vi "Bundle Test Graph Data.vi"(6 "ia test data":T1, 7 "diam time array in":dbl[](array[numeric]), 8 "setpoint array in":dbl[](array[numeric]), 9 "force array in":dbl[](array[numeric]), 10 "force time array in":dbl[](array[numeric]), 11 "diam array in":dbl[](array[numeric])) -> (0 "setpoint array out":dbl[](array[numeric]), 1 "force array out":dbl[](array[numeric]), 2 "force time array out":dbl[](array[numeric]), 3 "diam array out":dbl[](array[numeric]), 5 "diam time array out":dbl[](array[numeric]))   [LabVIEW 2020]
uses:
  Inflation Test/Result Handling/Inflation Test Numeric Results.ctl
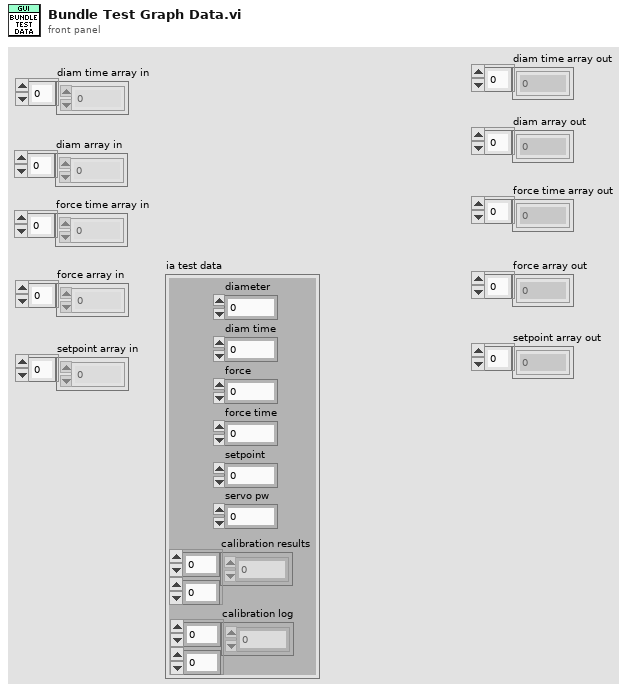
[diagram p1: front panel]
types:
  T1 = typedef "Inflation Test Numeric Results.ctl" = cluster{"diameter":dbl, "diam time":dbl, "force":dbl, "force time":dbl, "setpoint":dbl, "servo pw":dbl, "calibration log":dbl[][], "calibration results":dbl[][]}
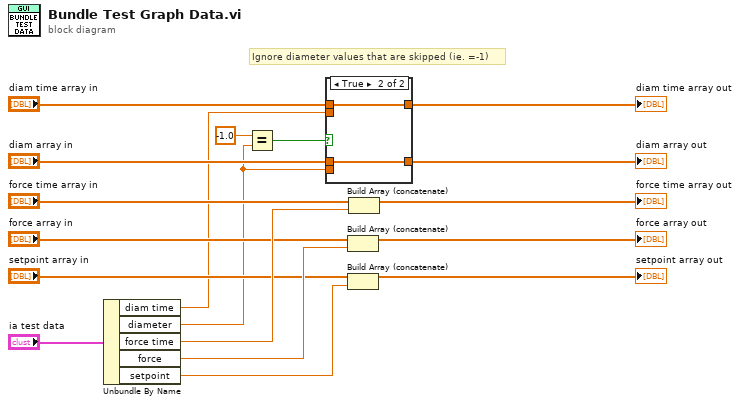
[diagram p0: block diagram]
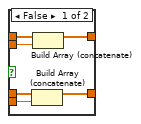
[diagram p2: hidden frame]
diagram:
  # "Ignore diameter values that are skipped (ie. =-1)"
  n1 = Unbundle By Name("ia test data") -> ("diam time"=w6:dbl, "diameter"=w3:dbl, "force time"=w11:dbl, "force"=w12:dbl, "setpoint"=w13:dbl)
  n2 = Equal?(x=-1.0, y=w3) -> (x = y?=w1:bool)
  n3 = case shown="True" w1 {
    tunnel: [w24 w25] -> w15
    tunnel: [w23 w26] -> w14
    tunnel: "diam array in" -> [w22 w25]
    tunnel: w6 -> [w21 _]
    tunnel: "diam time array in" -> [w20 w26]
    tunnel: w3 -> [w19 _]
    frame False {
      n4 = Build Array (concatenate)(w22, w19) -> (w24:dbl[])
      n5 = Build Array (concatenate)(w20, w21) -> (w23:dbl[])
    }
    frame True {
    }
  }
  "diam array out" <- w15
  "diam time array out" <- w14
  n6 = Build Array (concatenate)("force array in", w12) -> (→"force array out":dbl[])
  n7 = Build Array (concatenate)("setpoint array in", w13) -> (→"setpoint array out":dbl[])
  n8 = Build Array (concatenate)("force time array in", w11) -> (→"force time array out":dbl[])
